vi "Configure Trigger Model Digital Input Mode.vi"(8 "error in (no error)":errorcluster, 9 "Trigger Mode (Falling)":u16(ring) items=["Falling", "Rising", "Either"], 10 "Digital I/O line   (1)":i32=1 min=1 max=6 step=1 format="%#.6g", 11 "VISA resource name":refnum<visa-resource-name>) -> (0 "error out":errorcluster, 3 "VISA resource name out":refnum<visa-resource-name>)   [LabVIEW 2017, in "Keithley 2450.lvlib"]
doc: "This VI sets the logic on which the trigger event detector and the output trigger generator operate on the given trigger line."
uses:
  Keithley 2450.lvlib
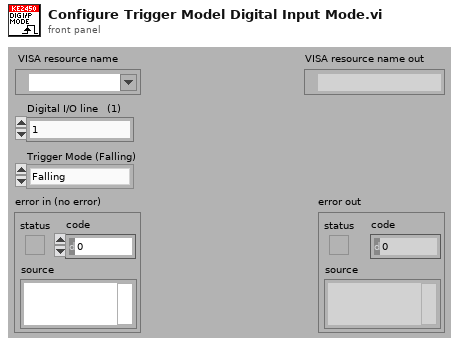
[diagram p1: front panel]
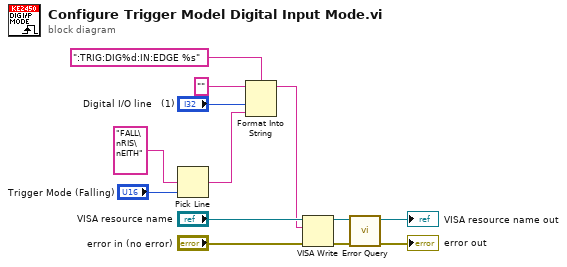
[diagram p0: block diagram]
diagram:
  n1 = Pick Line(multi-line string="FALL\nRIS\nEITH", line index="Trigger Mode (Falling)") -> (output string=w1:string)  [unwired: 1 in]
  n2 = Format Into String(format string=":TRIG:DIG%d:IN:EDGE %s", initial string="", "Digital I/O line   (1)", w1) -> (resulting string=w4:string)  [unwired: 1 in, 1 out]
  n3 = VISA Write(VISA resource name="VISA resource name", write buffer=w4, error in (no error)="error in (no error)") -> (VISA resource name out=w9:refnum<visa-resource-name>, error out=w8:errorcluster)  [unwired: 1 out]
  n4 = call "Error Query.vi"("error in (no error)"=w8, "VISA resource name"=w9) -> ("error out"=→"error out":errorcluster, "VISA resource name out"=→"VISA resource name out":refnum<visa-resource-name>)  [unwired: 8 out]
